vi "Agilent PWM Read Calibration Information.vi"(7 "Agilent PWM":T1, 8 "error in (no error)":errorcluster, 11 "VISA Resource Name":refnum<visa-resource-name>) -> (0 "error out":errorcluster, 1 "Calibration Due Date":timestamp, 2 "Calibration Date":timestamp, 3 "dup VISA Resource Name":refnum<visa-resource-name>)   [LabVIEW 2011]
uses:
  TypeDefs/Agilent PWM Instrument Info.ctl
  <vilib>/Utility/miscctls.llb/LVDateTimeRec.ctl
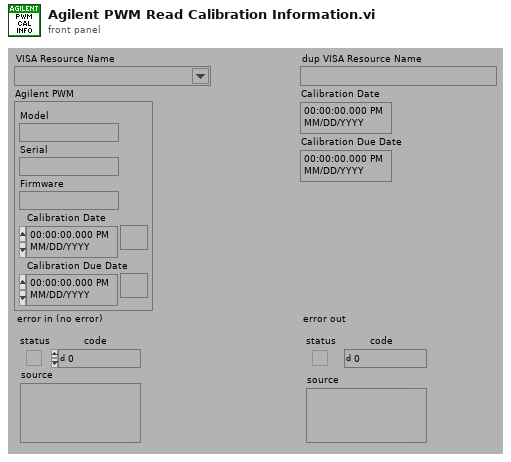
[diagram p1: front panel]
types:
  T1 = typedef "Agilent PWM Instrument Info.ctl" = cluster{"Model":string, "Serial":string, "Firmware":string, "Calibration Date":timestamp, "Calibration Due Date":timestamp}
  T2 = typedef "Agilent PWM Model.ctl" = enum16{"Not Supported", "E4418X", "E4419X", "U2000X"}
  T3 = typedef "LVDateTimeRec.ctl" = cluster{"fractional second":dbl, "second":i32, "minute":i32, "hour":i32, "day of month":i32, "month":i32, "year":i32, "day of week":i32, "day of year":i32, "DST":i32}
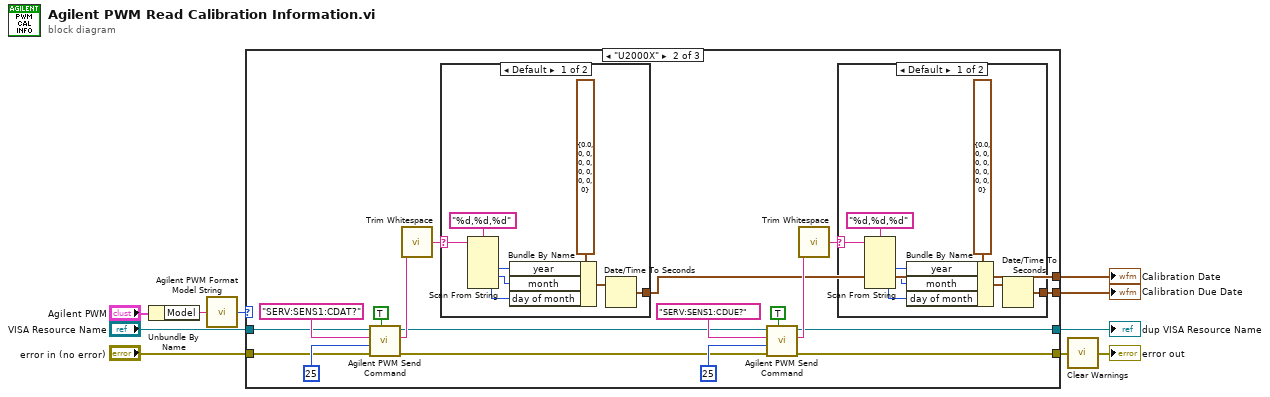
[diagram p0: block diagram]
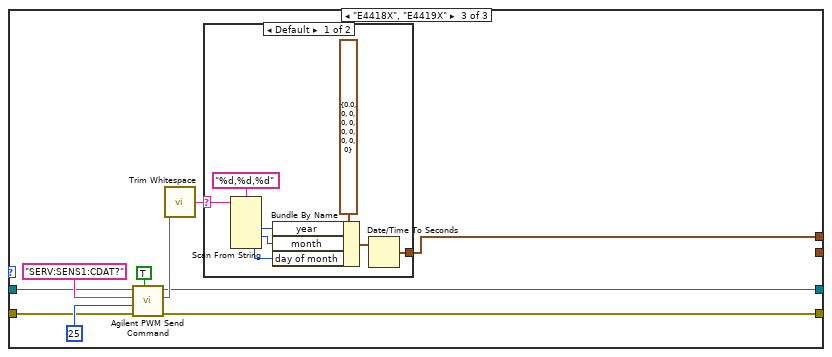
[diagram p5: hidden frame]
diagram:
  n1 = Unbundle By Name("Agilent PWM") -> ("Model"=w9:string)
  n2 = call "Agilent PWM Format Model String.vi"("Model"=w9) -> ("Model"=w8:T2)
  n3 = case shown="\"U2000X\"" w8 {
    tunnel: [w12 w15 w48] -> w10
    tunnel: "VISA Resource Name" -> [w11 w26 w52]
    tunnel: "error in (no error)" -> [w12 w25 w51]
    tunnel: [w11 w16 w49] -> w3
    tunnel: [_ w14 _] -> w2
    tunnel: [_ w13 w47] -> w1
    frame "Not Supported" {
    }
    frame "U2000X" {
      n4 = call "Agilent PWM Send Command.vi"("Read? (F)"=TRUE, "error in (no error)"=w25, "Byte Count"=u32 25, "Command"="SERV:SENS1:CDAT?" ("write buffer"), "VISA Resource Name"=w26) -> ("error out"=w17:errorcluster, "Data Read"=w27:string, "dup VISA Resource Name"=w18:refnum<visa-resource-name>)  [unwired: 4 out]
      n5 = call <vilib>:"Trim Whitespace.vi"("string"=w27) -> ("trimmed string"=w24:string)  [unwired: 1 in]
      n6 = case shown="Default" w24 {
        selector: w24 -> [w46 _]
        tunnel: [w39 _] -> w13
        frame Default {
          n7 = Scan From String(format string="%d,%d,%d", input string=w46) -> (output 1=w43:i32, output 2=w41:i32, output 3=w42:i32)  [unwired: 5 in, 3 out]
          n8 = Bundle By Name(cluster=T3 {"fractional second"=0.0, "second"=0, "minute"=0, "hour"=0, "day of month"=0, "month"=0, "year"=0, "day of week"=0, "day of year"=0, "DST"=0} ("date time rec"), "year"=w43, "month"=w41, "day of month"=w42) -> (w40:T3)
          n9 = Date/Time To Seconds(2:w40) -> (0:w39:timestamp)  [unwired: 1 in]
        }
        frame "NONE" {
        }
      }
      n10 = call "Agilent PWM Send Command.vi"("Read? (F)"=TRUE, "error in (no error)"=w17, "Byte Count"=u32 25, "Command"="SERV:SENS1:CDUE?" ("write buffer"), "VISA Resource Name"=w18) -> ("error out"=w15:errorcluster, "Data Read"=w22:string, "dup VISA Resource Name"=w16:refnum<visa-resource-name>)  [unwired: 4 out]
      n11 = call <vilib>:"Trim Whitespace.vi"("string"=w22) -> ("trimmed string"=w23:string)  [unwired: 1 in]
      n12 = case shown="Default" w23 {
        selector: w23 -> [w38 _]
        tunnel: [w31 _] -> w14
        frame Default {
          n13 = Scan From String(format string="%d,%d,%d", input string=w38) -> (output 1=w35:i32, output 2=w33:i32, output 3=w34:i32)  [unwired: 5 in, 3 out]
          n14 = Bundle By Name(cluster=T3 {"fractional second"=0.0, "second"=0, "minute"=0, "hour"=0, "day of month"=0, "month"=0, "year"=0, "day of week"=0, "day of year"=0, "DST"=0} ("date time rec"), "year"=w35, "month"=w33, "day of month"=w34) -> (w32:T3)
          n15 = Date/Time To Seconds(2:w32) -> (0:w31:timestamp)  [unwired: 1 in]
        }
        frame "NONE" {
        }
      }
    }
    frame "E4418X", "E4419X" {
      n16 = call "Agilent PWM Send Command.vi"("Read? (F)"=TRUE, "error in (no error)"=w51, "Byte Count"=u32 25, "Command"="SERV:SENS1:CDAT?" ("write buffer"), "VISA Resource Name"=w52) -> ("error out"=w48:errorcluster, "Data Read"=w53:string, "dup VISA Resource Name"=w49:refnum<visa-resource-name>)  [unwired: 4 out]
      n17 = call <vilib>:"Trim Whitespace.vi"("string"=w53) -> ("trimmed string"=w50:string)  [unwired: 1 in]
      n18 = case shown="Default" w50 {
        selector: w50 -> [w64 _]
        tunnel: [w57 _] -> w47
        frame Default {
          n19 = Scan From String(format string="%d,%d,%d", input string=w64) -> (output 1=w61:i32, output 2=w59:i32, output 3=w60:i32)  [unwired: 5 in, 3 out]
          n20 = Bundle By Name(cluster=T3 {"fractional second"=0.0, "second"=0, "minute"=0, "hour"=0, "day of month"=0, "month"=0, "year"=0, "day of week"=0, "day of year"=0, "DST"=0} ("date time rec"), "year"=w61, "month"=w59, "day of month"=w60) -> (w58:T3)
          n21 = Date/Time To Seconds(2:w58) -> (0:w57:timestamp)  [unwired: 1 in]
        }
        frame "NONE" {
        }
      }
    }
  }
  "dup VISA Resource Name" <- w3
  "Calibration Date" <- w1
  "Calibration Due Date" <- w2
  n22 = call "Clear Warnings.vi"("error in (no error)"=w10) -> ("error out"=→"error out":errorcluster)
